vi "Build.vi"(9 "XYZTheta":dbl[](array[numeric]), 10 "Pattern Coordinates":dbl[][](array[numeric]), 11 "C4 Dispense in":refnum<class "Iterative Dispense.lvclass">) -> (3 "C4 Dispense out":refnum<class "Iterative Dispense.lvclass">)   [LabVIEW 2020, in "Iterative Dispense.lvclass"]
uses:
  Iterative Dispense.lvclass
  Iterative Dispense.lvclass/Iterative Dispense.ctl
  <vilib>/Analysis/coordinate.llb/2D Cartesian Coordinate Rotation (Array).vi
  <vilib>/Analysis/NI_AALPro.lvlib
panel:
  out "array w/ subset deleted":dbl[][][](array[numeric])
  out "deleted portion":dbl[][](array[numeric])
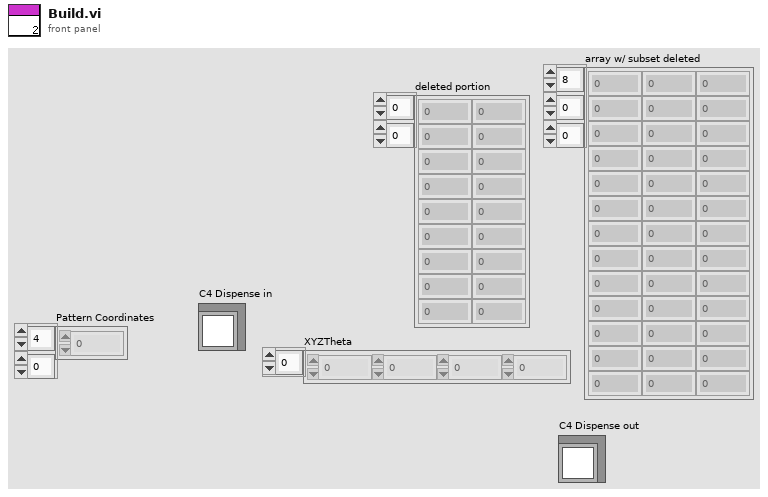
[diagram p1: front panel]
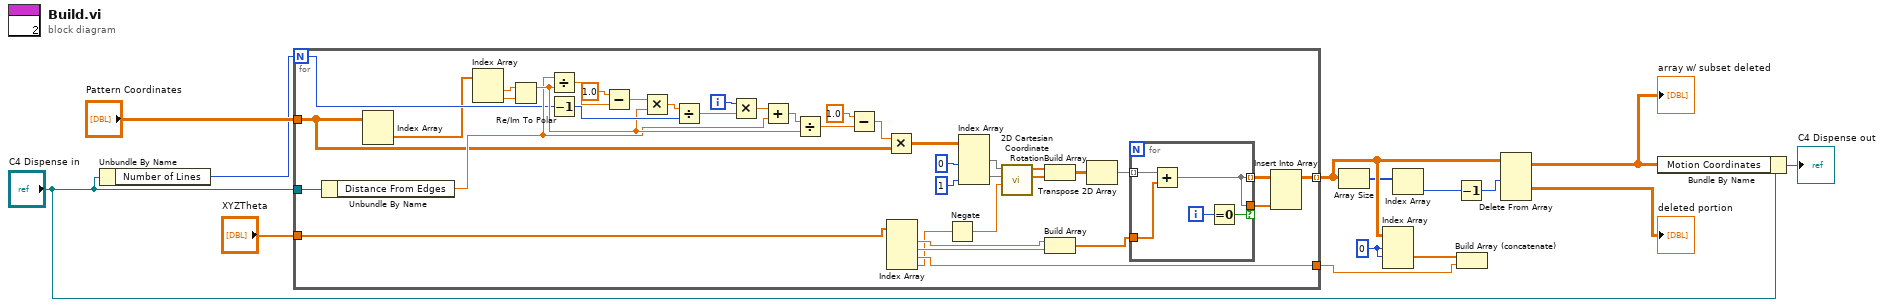
[diagram p0: block diagram]
diagram:
  w14 = 0 ("disabled index (page)")
  n1 = Unbundle By Name("C4 Dispense in") -> ("Number of Lines"=w9:i32)
  n2 = for {
    N: w9 -> [w29]
    tunnel: [w23] -> w5 mode=indexing
    tunnel: "XYZTheta" -> [w31]
    tunnel: "C4 Dispense in" -> [w35]
    tunnel: "Pattern Coordinates" -> [w22]
    tunnel: [w28] -> w11
    i -> [w48]
    n3 = Unbundle By Name(w35) -> ("Distance From Edges"=w34:dbl)
    n4 = Index Array(array=w22) -> (element=w21:dbl[])  [unwired: 2 in]
    n5 = Index Array(array=w21) -> (element #1=w20:dbl, element #2=w19:dbl)  [unwired: 2 in]
    n6 = Re/Im To Polar(2:w19, 3:w20) -> (1:w36:dbl)  [unwired: 1 out]
    n7 = Divide(x=w34, y=w36) -> (x/y=w42:dbl)
    n8 = Decrement(x=w29) -> (x-1=w38:i32)
    n9 = Subtract(x=1.0, y=w42) -> (x-y=w40:dbl)
    n10 = Multiply(x=w40, y=w36) -> (x*y=w39:dbl)
    n11 = Divide(x=w39, y=w38) -> (x/y=w37:dbl)
    n12 = Multiply(x=w48, y=w37) -> (x*y=w53:dbl)
    n13 = Add(x=w53, y=w34) -> (x+y=w52:dbl)
    n14 = Divide(x=w52, y=w36) -> (x/y=w51:dbl)
    n15 = Subtract(x=1.0, y=w51) -> (x-y=w43:dbl)
    n16 = Multiply(x=w43, y=w22) -> (x*y=w49:dbl[][])
    n17 = Index Array(array=w31) -> (element #1=w33:dbl, element #2=w32:dbl, element #3=w28:dbl, element #4=w16:dbl)  [unwired: 4 in]
    n18 = Negate(x=w16) -> (-x=w15:dbl)
    n19 = Index Array(array=w49, index (col) #1=0 ("disabled index (col)"), index (col) #2=1 ("index (col)")) -> (element #1=w27:dbl[], element #2=w26:dbl[])  [unwired: 2 in]
    n20 = call-poly <vilib>:"2D Cartesian Coordinate Rotation.vi"("theta"=w15, "Y"=w26, "X"=w27) -> ("Y Out"=w47:dbl[], "X Out"=w46:dbl[])  [unwired: 6 in, 1 out]
    n21 = Build Array(w46, w47) -> (w18:dbl[][])
    n22 = Build Array(w33, w32) -> (w30:dbl[])
    n23 = Transpose 2D Array(2D array=w18) -> (transposed array=w17:dbl[][])
    n24 = for {
      tunnel: w30 -> [w58]
      tunnel: w17 -> [w57] mode=indexing
      tunnel: [w54] -> w25 mode=indexing
      tunnel: [w54] -> w24 if=w55
      i -> [w56]
      n25 = Add(x=w57, y=w58) -> (x+y=w54:dbl[])
      n26 = Equal To 0?(x=w56) -> (x = 0?=w55:bool)
    }
    n27 = Insert Into Array(array=w25, new element=w24) -> (w23:dbl[][])  [unwired: 2 in]
  }
  n28 = Array Size(array=w5) -> (size(s)=w4:i32[])
  n29 = Index Array "Index Array"(array=w5, index (dim 0)=w14, index (dim 1)=w14) -> (element=w12:dbl[])  [unwired: 1 in]
  n30 = Index Array(array=w4) -> (element=w2:i32)  [unwired: 1 in]
  n31 = Decrement(x=w2) -> (x-1=w1:i32)
  n32 = Build Array (concatenate)(w12, w11) -> ()  [unwired: 1 out]
  n33 = Delete From Array "Delete From Array"(array=w5, index (dim 0)=w1) -> (deleted portion=→"deleted portion":dbl[][], array with subset deleted=w6:dbl[][][])  [unwired: 3 in]
  "array w/ subset deleted" <- w6
  n34 = Bundle By Name(cluster="C4 Dispense in", "Motion Coordinates"=w6) -> (→"C4 Dispense out":refnum<class "Iterative Dispense.lvclass">)
